vi "【抗扰】LADRC控制器-有节能函数.vi"() -> ()   [LabVIEW 2018]
panel:
  out "k进补偿LADRC":cluster{dbl, dbl}(graph)
  out "被减量":dbl
  in  "k":dbl(knob)=10.0 scale=0.0..40.0
  out "k进补偿LADRC":dbl
  out "温度":dbl(slide)=4.793814432989691 scale=0.0..250.0
  out "压力":dbl(slide)=0.6705882352941176 scale=0.0..1.0
  out "压力":T1(graph)
  out "温度":T2(graph)
  out "空气与蒸汽":dbl(slide)=0.49999999999999994 scale=0.0..1.0
  out "K进":dbl
  out "K排":dbl
  out "进气/排气":cluster{dbl, "上限":dbl}(graph)
  out "k空气":dbl
  out "k蒸汽":dbl
  out "z1 2":dbl
  out "z2 2":dbl
  out "z3 2":dbl
  out "u排":dbl
  in  "压力Pset":dbl=0.5
  out "压力":dbl
  in  "3P压力":cluster{"b0":dbl, "w0":dbl, "wc":dbl}={"b0"=40.0, "w0"=40.0, "wc"=150.0}
  in  "3P温度进气百分比":cluster{"b0":dbl, "w0":dbl, "wc":dbl}={"b0"=40.0, "w0"=40.0, "wc"=150.0}
  out "z1":dbl
  out "z2":dbl
  out "z3":dbl
  out "u":dbl
  in  "温度Tset":dbl=120.0
  out "dy/dt+z2":cluster{dbl, dbl}(graph)
  out "蒸汽/空气":cluster{dbl, "上限":dbl}(graph)
  out "温度":dbl
  out "排总":dbl(slide)=0.3 scale=0.0..100.0
  out "进总":dbl(slide)=0.5102040816326531 scale=0.0..100.0
  # "温度"
  # "蒸汽/空气"
  # "压力"
  # "进气/排气"
  # "温度\n/压力"
  # "+"
  # "R"
  # "kp"
  # "+"
  # "对象"
  # "u"
  # "+"
  # "1/b0"
  # "-"
  # "-"
  # "y"
  # "kd"
  # "z3"
  # "z2"
  # "线性扩张\n状态观测器"
  # "z1"
  # "LESO"
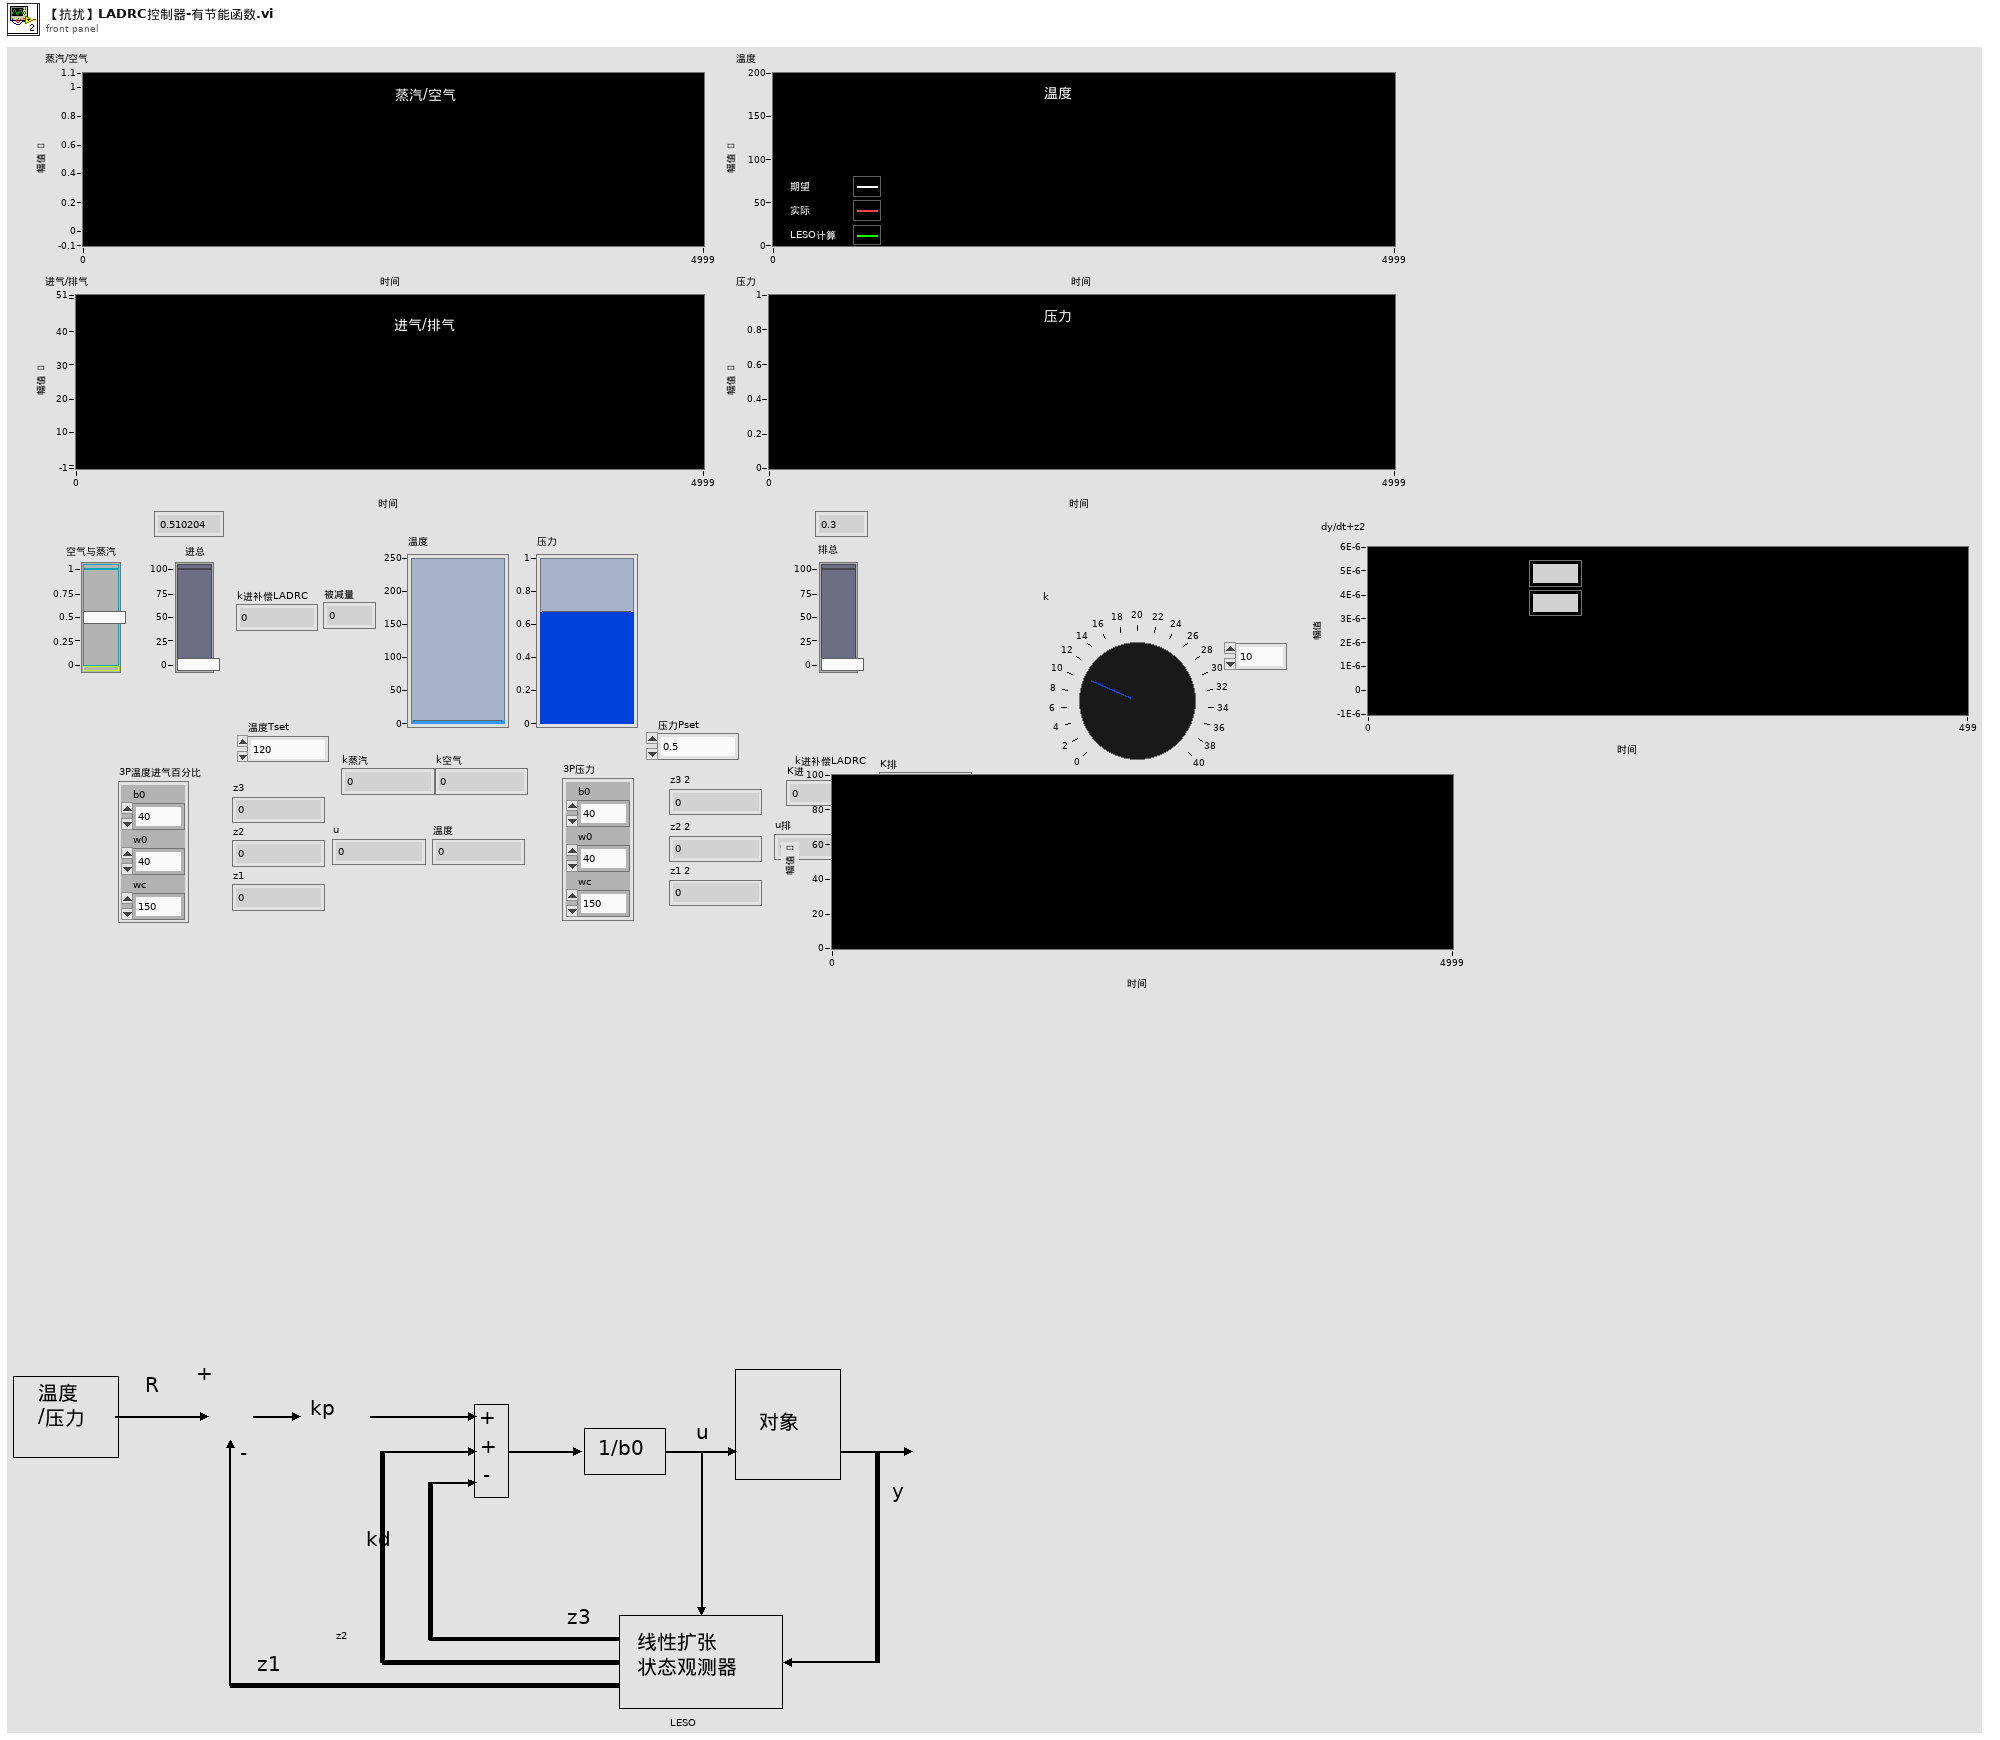
[diagram p1: front panel]
types:
  T1 = cluster{"压力Pset":dbl, "1M8仓压力仿真":dbl, "z1(k+1)":dbl}
  T2 = cluster{"温度Tset":dbl, "1M8仓温度仿真":dbl, "z1(k+1)":dbl}
  T3 = cluster{"温度Tset":dbl, "1M8仓温度仿真":dbl, "z1(k+1)":dbl}[]
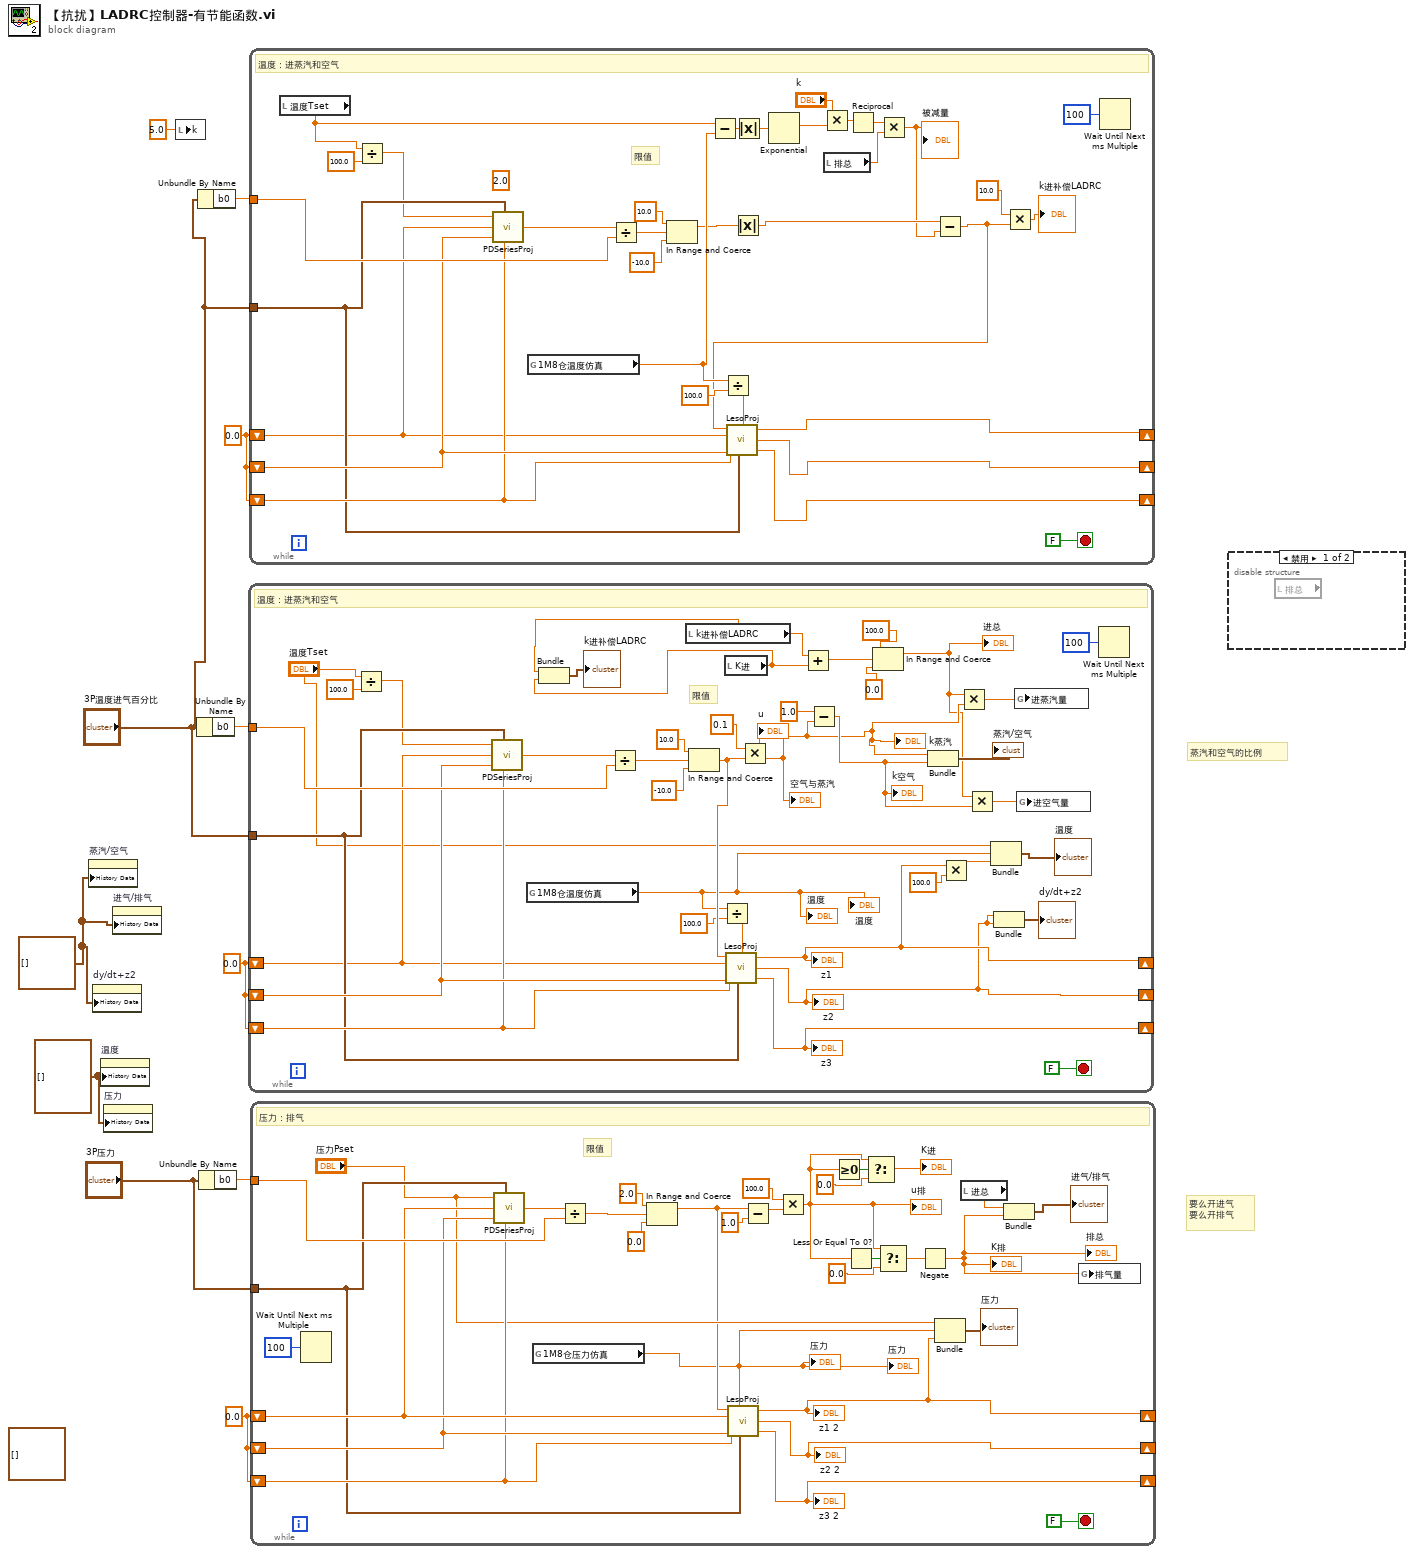
[diagram p0: block diagram]
diagram:
  w4 = 0.0 ("z1(k+1)")
  w6 = T3 [] ("历史数据")
  (unwired) cluster{dbl, dbl}[] [] ("历史数据")
  w7 = 0.0 ("z1(k+1)")
  w1 = cluster{dbl, dbl}[] [] ("历史数据")
  w11 = 0.0 ("z1(k+1)")
  # "要么开进气 \n要么开排气"
  # "蒸汽和空气的比例"
  n1 = property on="蒸汽/空气" class="WFChart (严格)"("History Data"=w1) -> ()  [unwired: 2 in, 2 out]
  n2 = property on="dy/dt+z2" class="WFChart (严格)"("History Data"=w1) -> ()  [unwired: 2 in, 2 out]
  n3 = property on="温度" class="WFChart (严格)"("History Data"=w6) -> ()  [unwired: 2 in, 2 out]
  n4 = property on="压力" class="WFChart (严格)"("History Data"=w6) -> ()  [unwired: 2 in, 2 out]
  n5 = property on="进气/排气" class="WFChart (严格)"("History Data"=w1) -> ()  [unwired: 2 in, 2 out]
  n6 = local write "k"(5.0 ("k")) -> ()
  n7 = Unbundle By Name("3P温度进气百分比") -> ("b0"=w10:dbl)
  n8 = Unbundle By Name("3P温度进气百分比") -> ("b0"=w5:dbl)
  n9 = Unbundle By Name("3P压力") -> ("b0"=w8:dbl)
  n10 = while {
    tunnel: w10 -> [w49]
    shift-right: [w26] -> _
    shift-left: w11 -> [w33]
    shift-right: [w15] -> _
    shift-left: w11 -> [w43]
    shift-right: [w48] -> _
    shift-left: w11 -> [w42]
    tunnel: "3P温度进气百分比" -> [w40]
    stop <- FALSE stop-if-true
    # "限值"
    # "温度：进蒸汽和空气"
    n11 = Divide(x="温度Tset", y=100.0) -> (x/y=w32:dbl)
    n12 = call "PDSeriesProj.vi"("Input"=w32, "3Parameter"=w40, "Z1"=w33, "Z2"=w43, "Z3"=w42) -> ("U0-Z3"=w41:dbl)
    n13 = global read "全局变量.vi" "1M8仓温度仿真"() -> (w16:dbl)
    "温度" <- w16
    "温度" <- w16
    n14 = Divide(x=w41, y=w49) -> (x/y=w46:dbl)
    n15 = local read "k进补偿LADRC"() -> (w13:dbl)
    n16 = In Range and Coerce(upper limit=10.0 ("上限"), x=w46, lower limit=-10.0 ("下限")) -> (coerced(x)=w34:dbl)  [unwired: 1 out]
    n17 = Divide(x=w16, y=100.0) -> (x/y=w30:dbl)
    n18 = local read "K进"() -> (w12:dbl)
    n19 = Bundle("k进补偿LADRC"=w13, "K进"=w12) -> (→"k进补偿LADRC":cluster{"k进补偿LADRC":dbl, "K进":dbl})  [unwired: 1 in]
    n20 = call "LesoProj.vi"("u"=w34, "y"=w30, "z1(k)"=w33, "z3(k)"=w42, "3Parameter"=w40, "z2(k)"=w43) -> ("z1(k+1)"=w26:dbl, "z2(k+1)"=w15:dbl, "z3(k+1)"=w48:dbl)
    "z1" <- w26
    "z2" <- w15
    "z3" <- w48
    n21 = Multiply(x=0.1, y=w34) -> (x*y=w24:dbl)
    "u" <- w24
    "k蒸汽" <- w24
    "空气与蒸汽" <- w24
    n22 = Add(x=w13, y=w12) -> (x+y=w17:dbl)
    n23 = Subtract(x=1.0, y=w24) -> (x-y=w35:dbl)
    "k空气" <- w35
    n24 = In Range and Coerce(upper limit=100.0 ("上限"), x=w17, lower limit=0.0 ("下限")) -> (coerced(x)=w20:dbl)  [unwired: 1 out]
    "进总" <- w20
    n25 = Bundle(w24, w35) -> (→"蒸汽/空气":cluster{dbl, dbl})  [unwired: 1 in]
    n26 = Multiply(x=w26, y=100.0) -> (x*y=w27:dbl)
    n27 = Multiply(x=w20, y=w24) -> (x*y=w22:dbl)
    n28 = Multiply(x=w20, y=w35) -> (x*y=w21:dbl)
    n29 = Bundle("温度Tset"="温度Tset", "1M8仓温度仿真"=w16, w27) -> (→"温度":cluster{"温度Tset":dbl, "1M8仓温度仿真":dbl, dbl})  [unwired: 1 in]
    n30 = Bundle("z2(k+1)"=w15, "z2(k+1)"=w15) -> (→"dy/dt+z2":cluster{"z2(k+1)":dbl, "z2(k+1)":dbl})  [unwired: 1 in]
    n31 = global write "全局变量.vi" "进蒸汽量"(w22) -> ()
    n32 = global write "全局变量.vi" "进空气量"(w21) -> ()
    n33 = Wait Until Next ms Multiple(millisecond multiple=u32 100 ("毫秒倍数")) -> ()  [unwired: 1 out]
  }
  n34 = while {
    tunnel: w5 -> [w82]
    shift-right: [w66] -> _
    shift-left: w4 -> [w71]
    shift-right: [w72] -> _
    shift-left: w4 -> [w77]
    shift-right: [w81] -> _
    shift-left: w4 -> [w76]
    tunnel: "3P温度进气百分比" -> [w74]
    stop <- FALSE stop-if-true
    (unwired) 2.0 ("y")
    # "限值"
    # "温度：进蒸汽和空气"
    n35 = local read "温度Tset"() -> (w64:dbl)
    n36 = Divide(x=w64, y=100.0) -> (x/y=w70:dbl)
    n37 = call "PDSeriesProj.vi"("Input"=w70, "3Parameter"=w74, "Z1"=w71, "Z2"=w77, "Z3"=w76) -> ("U0-Z3"=w75:dbl)
    n38 = global read "全局变量.vi" "1M8仓温度仿真"() -> (w63:dbl)
    n39 = Divide(x=w75, y=w82) -> (x/y=w80:dbl)
    n40 = In Range and Coerce(upper limit=10.0 ("上限"), x=w80, lower limit=-10.0 ("下限")) -> (coerced(x)=w61:dbl)  [unwired: 1 out]
    n41 = Subtract(x=w64, y=w63) -> (x-y=w62:dbl)
    n42 = Divide(x=w63, y=100.0) -> (x/y=w68:dbl)
    n43 = Absolute Value(x=w61) -> (abs(x)=w54:dbl)
    n44 = Absolute Value(x=w62) -> (abs(x)=w57:dbl)
    n45 = Exponential(1:w57) -> (0:w58:dbl)
    n46 = Multiply(x="k", y=w58) -> (x*y=w55:dbl)
    n47 = local read "排总"() -> (w59:dbl)
    n48 = Reciprocal(x=w55) -> (1/x=w60:dbl)
    n49 = Multiply(x=w60, y=w59) -> (x*y=w51:dbl)
    "被减量" <- w51
    n50 = Subtract(x=w54, y=w51) -> (x-y=w52:dbl)
    n51 = call "LesoProj.vi"("u"=w52, "y"=w68, "z1(k)"=w71, "z3(k)"=w76, "3Parameter"=w74, "z2(k)"=w77) -> ("z1(k+1)"=w66:dbl, "z2(k+1)"=w72:dbl, "z3(k+1)"=w81:dbl)
    n52 = Multiply(x=10.0, y=w52) -> (x*y=→"k进补偿LADRC":dbl)
    n53 = Wait Until Next ms Multiple(millisecond multiple=u32 100 ("毫秒倍数")) -> ()  [unwired: 1 out]
  }
  n54 = while {
    tunnel: w8 -> [w113]
    shift-right: [w112] -> _
    shift-left: w7 -> [w108]
    shift-right: [w102] -> _
    shift-left: w7 -> [w107]
    shift-right: [w111] -> _
    shift-left: w7 -> [w106]
    tunnel: "3P压力" -> [w104]
    stop <- FALSE stop-if-true
    # "限值"
    # "压力：排气"
    n55 = Wait Until Next ms Multiple(millisecond multiple=u32 100 ("毫秒倍数")) -> ()  [unwired: 1 out]
    n56 = call "PDSeriesProj.vi"("Input"="压力Pset", "3Parameter"=w104, "Z1"=w108, "Z2"=w107, "Z3"=w106) -> ("U0-Z3"=w105:dbl)
    n57 = global read "全局变量.vi" "1M8仓压力仿真"() -> (w85:dbl)
    "压力" <- w85
    "压力" <- w85
    n58 = Divide(x=w105, y=w113) -> (x/y=w90:dbl)
    n59 = In Range and Coerce(upper limit=2.0 ("上限"), x=w90, lower limit=0.0 ("下限")) -> (coerced(x)=w93:dbl)  [unwired: 1 out]
    n60 = call "LesoProj.vi"("u"=w93, "y"=w85, "z1(k)"=w108, "z3(k)"=w106, "3Parameter"=w104, "z2(k)"=w107) -> ("z1(k+1)"=w112:dbl, "z2(k+1)"=w102:dbl, "z3(k+1)"=w111:dbl)
    "z1 2" <- w112
    "z2 2" <- w102
    "z3 2" <- w111
    n61 = Subtract(x=w93, y=1.0) -> (x-y=w87:dbl)
    n62 = Multiply(x=100.0, y=w87) -> (x*y=w89:dbl)
    "u排" <- w89
    n63 = Greater Or Equal To 0?(x=w89) -> (x >= 0?=w98:bool)
    n64 = Less Or Equal To 0?(x=w89) -> (x <= 0?=w95:bool)
    n65 = Select(t=w89, s=w98, f=0.0) -> (s? t:f=→"K进":dbl)
    n66 = Select(t=w89, s=w95, f=0.0) -> (s? t:f=w94:dbl)
    n67 = Negate(x=w94) -> (-x=w91:dbl)
    "K排" <- w91
    "排总" <- w91
    n68 = Bundle("压力Pset"="压力Pset", "1M8仓压力仿真"=w85, "z1(k+1)"=w112) -> (→"压力":T1)  [unwired: 1 in]
    n69 = local read "进总"() -> (w84:dbl)
    n70 = Bundle("进总"=w84, w91) -> (→"进气/排气":cluster{"进总":dbl, dbl})  [unwired: 1 in]
    n71 = global write "全局变量.vi" "排气量"(w91) -> ()
  }
  n72 = disable-structure shown="禁用" {
    frame Disabled {
      n73 = local read "排总"() -> ()  [unwired: 1 out]
    }
    frame Enabled {
    }
  }
